vi "Dz Zero Function.vi"(4 "data":variant, 5 "x":dbl) -> (2 "f(x)":dbl)   [LabVIEW 2014]
doc: "Function for finding the mobility diameter <B>x</B> given the mobility, number of charges on the particle <B>n</B> and the mobility <B>Z1</B>."
uses:
  DMA Data.ctl
  Atmospheric/Atmospheric Constants.vi
  Atmospheric/Atmospheric Library.lvlib
  DMA.lvclass
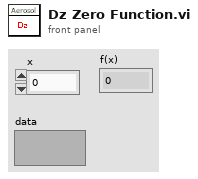
[diagram p1: front panel]
types:
  T1 = typedef "DMA.lvclass/DMA Data.ctl" = cluster{"T":dbl, "P":dbl, "n":i32, "mu":dbl, "Z1":dbl}
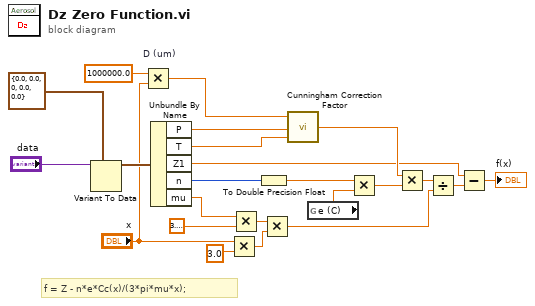
[diagram p0: block diagram]
diagram:
  # "f = Z - n*e*Cc(x)/(3*pi*mu*x);"
  n1 = Variant To Data(type=T1 {"T"=0.0, "P"=0.0, "n"=0, "mu"=0.0, "Z1"=0.0}, Variant="data") -> (data=w12:T1)  [unwired: 1 in, 1 out]
  n2 = Multiply "D (um)"(x=1000000.0, y="x") -> (x*y=w6:dbl)
  n3 = Unbundle By Name(w12) -> ("P"=w2:dbl, "T"=w3:dbl, "Z1"=w1:dbl, "n"=w5:i32, "mu"=w11:dbl)
  n4 = Multiply(x="x", y=3.0) -> (x*y=w17:dbl)
  n5 = Multiply(x=w11, y=3.141592653589793) -> (x*y=w18:dbl)
  n6 = To Double Precision Float(number=w5) -> (double precision float=w4:dbl)
  n7 = Multiply(x=w18, y=w17) -> (x*y=w15:dbl)
  n8 = call "Cunningham Correction Factor.vi"("T (K)"=w3, "P (mb)"=w2, "D (mm)"=w6) -> ("Cc"=w22:dbl)
  n9 = global read "Atmospheric Constants.vi" "e (C)"() -> (w23:dbl)
  n10 = Multiply(x=w4, y=w23) -> (x*y=w21:dbl)
  n11 = Multiply(x=w22, y=w21) -> (x*y=w16:dbl)
  n12 = Divide(x=w16, y=w15) -> (x/y=w14:dbl)
  n13 = Subtract(x=w1, y=w14) -> (x-y=→"f(x)":dbl)
